vi "Auto adjust sensitivity.vi"(0 "Lockin SR830 in":refnum<class "Lockin SR830.lvclass">, 7 "R value":dbl format="%#_13g", 9 "Input Setting":i32, 11 "error in (no error)":errorcluster) -> (4 "Lockin SR830 out":refnum<class "Lockin SR830.lvclass">, 10 "Repeat Measurement?":bool, 15 "error out":errorcluster)   [LabVIEW 2023, in "Lockin SR830.lvclass"]
uses:
  Lockin SR830.lvclass
  Lockin SR830.lvclass/Lockin SR830.ctl
  sr830/SR830.lvlib
panel:
  in  "Post Adjust Wait":dbl[unit]=0.1
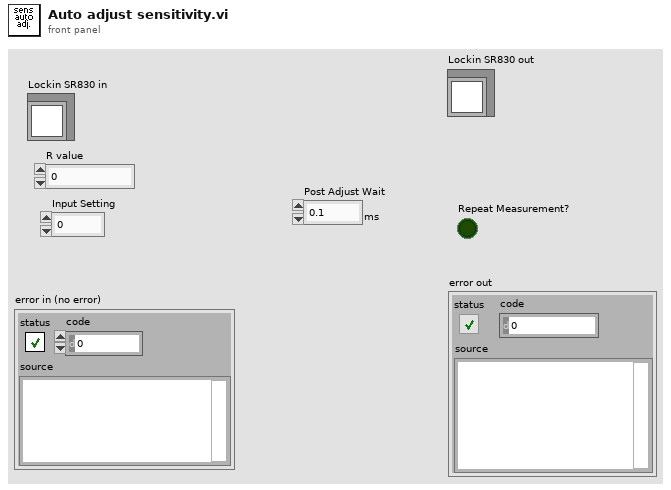
[diagram p1: front panel]
types:
  T1 = typedef "Lockin SR830.lvclass/Sensitivity.ctl" = u16
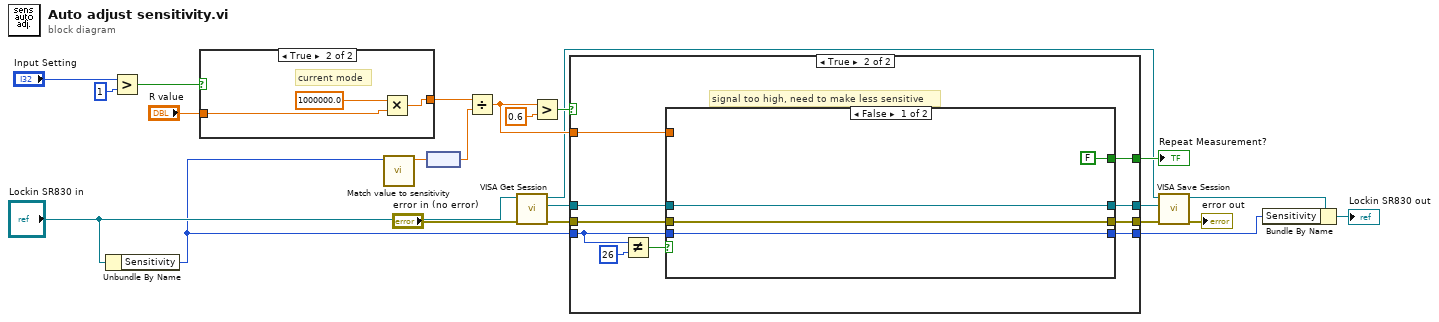
[diagram p0: block diagram]
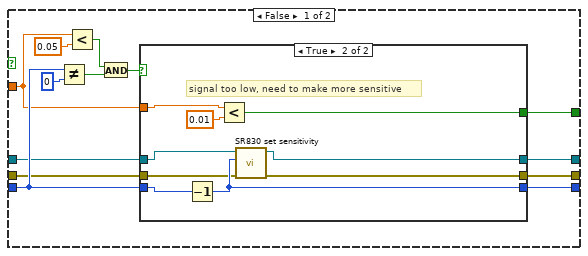
[diagram p2: hidden frame]
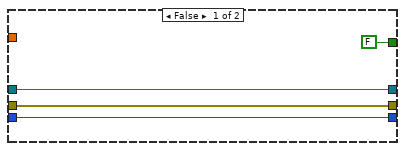
[diagram p3: hidden frame]
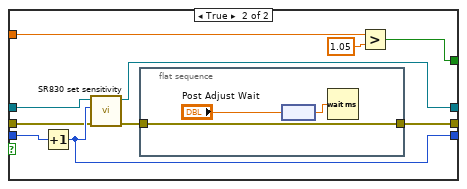
[diagram p4: hidden frame]
diagram:
  n1 = Unbundle By Name("Lockin SR830 in") -> ("Sensitivity"=w4:T1)
  n2 = Greater?(x="Input Setting", y=1) -> (0:w21:bool)
  n3 = case shown="True" w21 {
    tunnel: "R value" -> [w24 w26]
    tunnel: [w24 w25] -> w17
    frame False {
      # "voltage mode"
    }
    frame True {
      # "current mode"
      n4 = Multiply(x=1000000.0, y=w26) -> (x*y=w25:dbl)
    }
  }
  n5 = call "Match value to sensitivity.vi"("integer"=w4) -> ("sensitivity"=w14:dbl[unit])  [unwired: 10 in]
  n6 = node(w14) -> (w15:dbl)
  n7 = Divide(x=w17, y=w15) -> (x/y=w18:dbl)
  n8 = call-dynamic "VISA Get Session.vi"("error in (no error)"="error in (no error)", "Instrument.lvclass in"="Lockin SR830 in") -> ("error out"=w6:errorcluster, "VISA Resource Name"=w12:refnum<visa-resource-name>, "Instrument.lvclass out"=w8:refnum<class "Lockin SR830.lvclass">)  [unwired: 7 out]
  n9 = Greater?(x=w18, y=0.6) -> (0:w19:bool)
  n10 = case shown="True" w19 {
    tunnel: w4 -> [w36 w61]
    tunnel: w18 -> [w30 w60]
    tunnel: w12 -> [w34 w59]
    tunnel: [w35 w58] -> w10
    tunnel: [w32 w57] -> w2
    tunnel: [w31 w56] -> w13
    tunnel: [w29 w55] -> w11
    tunnel: w6 -> [w28 w54]
    frame False {
      n11 = Not Equal?(x=w36, y=0) -> (x != y?=w37:bool)
      n12 = Less?(x=w30, y=0.05) -> (x < y?=w38:bool)
      n13 = And(x=w38, y=w37) -> (x .and. y?=w33:bool)
      n14 = case shown="True" w33 {
        tunnel: w36 -> [w43 w53]
        tunnel: w28 -> [w44 w51]
        tunnel: [w44 w45] -> w35
        tunnel: w34 -> [w41 w50]
        tunnel: [w43 w52] -> w32
        tunnel: [FALSE w47] -> w31
        tunnel: w30 -> [_ w49]
        tunnel: [w41 w46] -> w29
        frame False {
        }
        frame True {
          # "signal too low, need to make more sensitive"
          n15 = Decrement(x=w53) -> (x-1=w52:T1)
          n16 = Less?(x=w49, y=0.01) -> (x < y?=w47:bool)
          n17 = call "SR830 set sensitivity.vi"("error in (no error)"=w51, "Sensitivity"=w52, "VISA resource name"=w50) -> ("error out"=w45:errorcluster, "VISA resource name out"=w46:refnum<visa-resource-name>)  [unwired: 7 in]
        }
      }
    }
    frame True {
      # "signal too high, need to make less sensitive"
      n18 = Not Equal?(x=w61, y=26) -> (x != y?=w62:bool)
      n19 = case shown="False" w62 {
        tunnel: w61 -> [w66 w77]
        tunnel: w60 -> [_ w76]
        tunnel: [FALSE w74] -> w56
        tunnel: w59 -> [w65 w72]
        tunnel: [w64 w73] -> w58
        tunnel: [w66 w71] -> w57
        tunnel: [w65 w70] -> w55
        tunnel: w54 -> [w64 w68]
        frame False {
        }
        frame True {
          n20 = Increment(x=w77) -> (x+1=w71:T1)
          n21 = call "SR830 set sensitivity.vi"("error in (no error)"=w68, "Sensitivity"=w71, "VISA resource name"=w72) -> ("error out"=w69:errorcluster, "VISA resource name out"=w70:refnum<visa-resource-name>)  [unwired: 7 in]
          n22 = flat-sequence {
            tunnel: [w79] -> w73
            tunnel: w69 -> [w79]
            frame #0 {
              n23 = node("Post Adjust Wait") -> (w78:dbl)
              n24 = Wait (ms)(milliseconds to wait=w78) -> ()  [unwired: 1 out]
            }
          }
          n25 = Greater?(x=w76, y=1.05) -> (0:w74:bool)
        }
      }
    }
  }
  "Repeat Measurement?" <- w13
  n26 = call-dynamic "VISA Save Session.vi"("error in (no error)"=w10, "VISA Resource Name"=w11, "Instrument.lvclass in"=w8) -> ("error out"=→"error out":errorcluster, "Instrument.lvclass out"=w3:refnum<class "Lockin SR830.lvclass">)  [unwired: 7 out]
  n27 = Bundle By Name(cluster=w3, "Sensitivity"=w2) -> (→"Lockin SR830 out":refnum<class "Lockin SR830.lvclass">)
